vi "MoveSampleAndSave.vi"(4 "Offset (V)":dbl, 5 "Total Y-axis Distance (mm)":dbl, 6 "x (in units of D)":i32=1, 7 "File Save Path":string="C:\\Users\\Carlos\\Documents\\Garcia_Carlos", 8 "Y Calibration Constant":dbl, 9 "Y-axis Distance/Sample":dbl, 10 "Axis#":i16 min=0 max=2 step=1, 11 "Forward/Reverse":bool) -> ()   [LabVIEW 2017]
uses:
  <vilib>/Analysis/baseanly.llb/Mean (DBL).vi
  <vilib>/Analysis/NI_AALBase.lvlib
panel:
  out "5V Indicator":bool
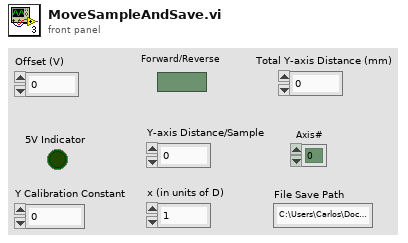
[diagram p1: front panel]
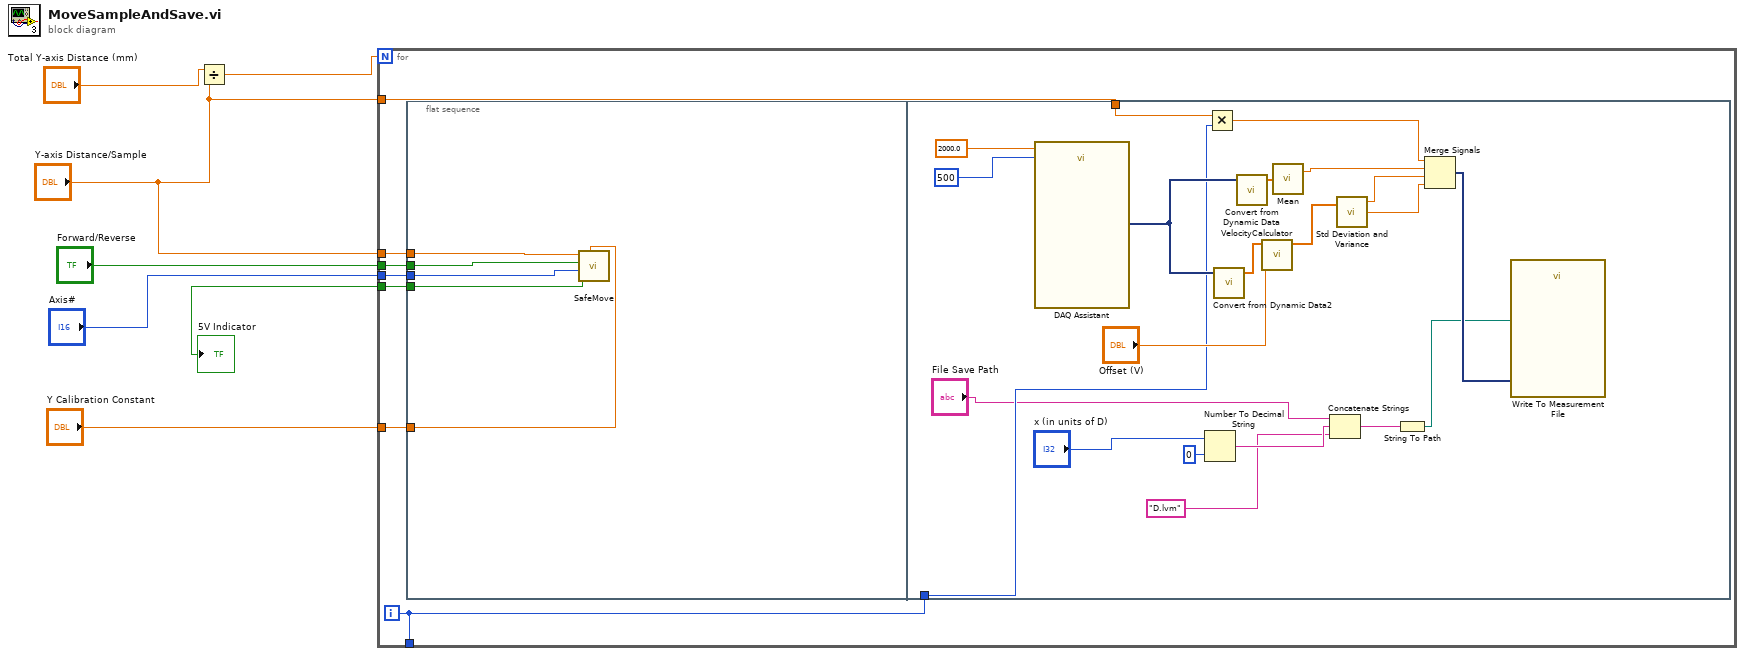
[diagram p0: block diagram]
diagram:
  n1 = Divide(x="Total Y-axis Distance (mm)", y="Y-axis Distance/Sample") -> (x/y=w4:dbl)
  n2 = for {
    N: w4 -> [_]
    tunnel: "Forward/Reverse" -> [w14]
    tunnel: "Axis#" -> [w13]
    tunnel: "Y-axis Distance/Sample" -> [w12]
    tunnel: [w10] -> _
    tunnel: "Y-axis Distance/Sample" -> [w11]
    tunnel: [w9] -> w2
    tunnel: "Y Calibration Constant" -> [w8]
    i -> [w10]
    n3 = flat-sequence {
      tunnel: w14 -> [w18]
      tunnel: w13 -> [w17]
      tunnel: w12 -> [w19]
      tunnel: [w16] -> w9
      tunnel: w8 -> [w15]
      tunnel: w11 -> [w27]
      tunnel: w10 -> [w26]
      frame #0 {
        n4 = call "SafeMove.vi"("Calibration Constant"=w15, "Axis#"=w17, "Forward/Reverse"=w18, "Total Distance (mm)"=w19) -> ("5V Indicator"=w16:bool)  [unwired: 7 in]
      }
      frame #1 {
        n5 = call "DAQ Assistant"("rate"=2000.0, "number of samples"=500) -> ("data"=w39:dynamicdata)  [unwired: 15 in, 2 out]
        n6 = Number To Decimal String(number="x (in units of D)", width (-)=i16 0) -> (decimal integer string=w32:string)
        n7 = Multiply(x=w27, y=w26) -> (x*y=w28:dbl)
        n8 = call "Convert from Dynamic Data2"("Dynamic Data Type"=w39) -> ("Array"=w38:dbl[])  [unwired: 3 in]
        n9 = call "Convert from Dynamic Data"("Dynamic Data Type"=w39) -> ("Array"=w40:dbl[])  [unwired: 3 in]
        n10 = call "VelocityCalculator.vi"("Offset (V)"="Offset (V)", "Voltage Input"=w38) -> ("Veloctiy Output [m/s]"=w24:dbl[])  [unwired: 9 in]
        n11 = call-poly <vilib>:"Mean.vi"("X"=w40) -> ("mean"=w36:dbl)  [unwired: 1 out]
        n12 = Concatenate Strings("File Save Path", w32, "D.lvm" ("string")) -> (w34:string)
        n13 = call <vilib>:"Std Deviation and Variance.vi"("X"=w24) -> ("mean"=w23:dbl, "standard deviation"=w22:dbl)  [unwired: 1 in, 1 out]
        n14 = String To Path(string=w34) -> (path=w33:path)
        n15 = Merge Signals(w28, w36, w23, w22) -> (w35:dynamicdata)
        n16 = call "Write To Measurement File"("Signals"=w35, "Filename"=w33) -> ()  [unwired: 15 in, 3 out]
      }
    }
  }
  "5V Indicator" <- w2
